vi "rx streamer issue stream cmd.vi"(8 "error in (no error)":errorcluster, 10 "stream_cmd":T1={"stream_mode"=97, "@dummy control@"=0, "@dummy control@"=0, "@dummy control@"=0, "@dummy control@"=0, "num_samps"=0, "stream_now"=0, "@dummy control@"=0, "@dummy control@"=0, "@dummy control@"=0, "@dummy control@"=0, "time_spec_full_secs"=0, "time_spec_frac_secs"=0.0} {"stream_mode" items=["UHD_STREAM_MODE_START_CONTINUOUS"=97, "UHD_STREAM_MODE_STOP_CONTINUOUS"=111, "UHD_STREAM_MODE_NUM_SAMPS_AND_DONE"=100, "UHD_STREAM_MODE_NUM_SAMPS_AND_MORE"=109]}, 11 "h":u64) -> (0 "error out":errorcluster, 2 "function return":u32(ring), 3 "h 2":u64)   [LabVIEW 2023, in "uhd.lvlib"]
doc: "UHD_API uhd_error uhd_rx_streamer_issue_stream_cmd(\n uhd_rx_streamer_handle h, const uhd_stream_cmd_t* stream_cmd);"
uses:
  <userlib>/uhd/uhd.lvlib
  <userlib>/uhd/uhd.dll
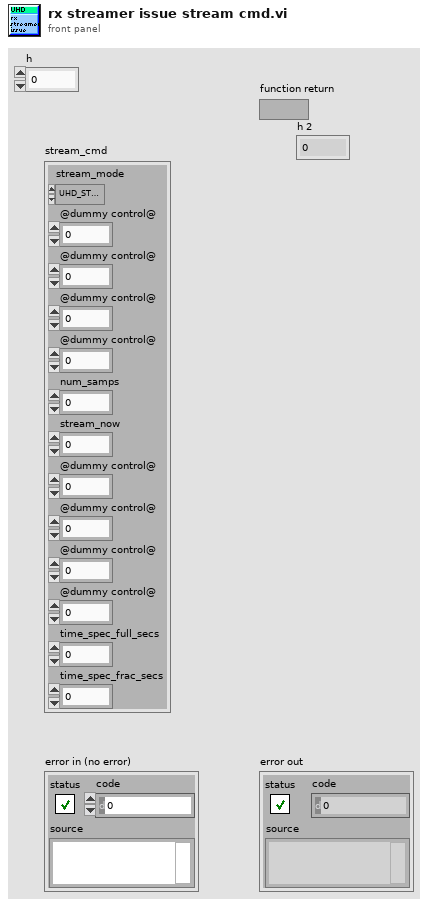
[diagram p1: front panel]
types:
  T1 = cluster{"stream_mode":u32, "@dummy control@":i8, "@dummy control@":i8, "@dummy control@":i8, "@dummy control@":i8, "num_samps":u64, "stream_now":i32, "@dummy control@":i8, "@dummy control@":i8, "@dummy control@":i8, "@dummy control@":i8, "time_spec_full_secs":i64, "time_spec_frac_secs":dbl}
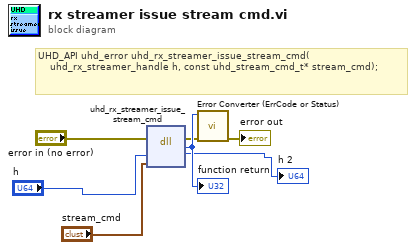
[diagram p0: block diagram]
diagram:
  # "UHD_API uhd_error uhd_rx_streamer_issue_stream_cmd(\n    uhd_rx_streamer_handle h, const uhd_stream_cmd_t* stream_cmd);"
  n1 = dll-call lib="C:/Program Files/National Instruments/LabVIEW 2023/user.lib/uhd/uhd.*" fn="uhd_rx_streamer_issue_stream_cmd"(error in="error in (no error)", "h"="h", "stream_cmd"="stream_cmd") -> (error out=w4:errorcluster, w7:u32, "h"=→"h 2":u64)  [unwired: 3 in, 1 out]
  "function return" <- w7
  n2 = call <userlib>:"Error Converter (ErrCode or Status).vi"("error in (no error)"=w4, "error code"=w7) -> ("error out"=→"error out":errorcluster)  [unwired: 9 in]
